vi "Move the peace.vi"(9 "Move Right":bool, 10 "Stack Array":u8[][](array[numeric]), 11 "Piece Array":u8[][](array[numeric])) -> (3 "Moved Piece Array":u8[][](array[numeric]))   [LabVIEW 2019]
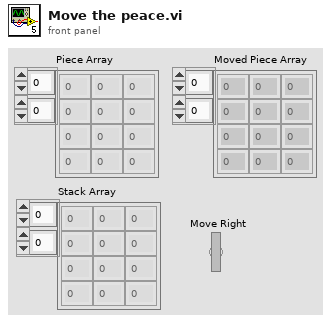
[diagram p1: front panel]
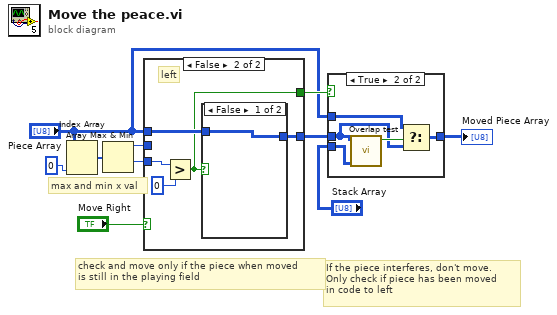
[diagram p0: block diagram]
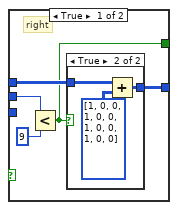
[diagram p3: hidden frame]
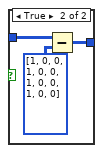
[diagram p5: hidden frame]
diagram:
  # "max and min x val"
  # "If the piece interferes, don't move.\nOnly check if piece has been moved \nin code to left"
  # "check and move only if the piece when moved\nis still in the playing field"
  n1 = Index Array(array="Piece Array", index (col)=0) -> (element=w10:u8[])  [unwired: 1 in]
  n2 = Array Max & Min(array=w10) -> (max value=w8:u8, min value=w1:u8)  [unwired: 2 out]
  n3 = case shown="False" "Move Right" {
    tunnel: w8 -> [w15 _]
    tunnel: "Piece Array" -> [w13 w23]
    tunnel: [w12 w22] -> w6
    tunnel: [w11 w21] -> w5
    tunnel: w1 -> [_ w20]
    frame True {
      # "right"
      n4 = Less?(x=w15, y=9) -> (x < y?=w12:bool)
      n5 = case shown="True" w12 {
        tunnel: w13 -> [w16 w18]
        tunnel: [w16 w17] -> w11
        frame False {
        }
        frame True {
          n6 = Add(x=w18, y=i32[][] [[1, 0, 0], [1, 0, 0], [1, 0, 0], [1, 0, 0]]) -> (x+y=w17:i32[][])
        }
      }
    }
    frame False {
      # "left"
      n7 = Greater?(x=w20, y=0) -> (0:w22:bool)
      n8 = case shown="False" w22 {
        tunnel: w23 -> [w25 w27]
        tunnel: [w25 w26] -> w21
        frame False {
        }
        frame True {
          n9 = Subtract(x=w27, y=i32[][] [[1, 0, 0], [1, 0, 0], [1, 0, 0], [1, 0, 0]]) -> (x-y=w26:i32[][])
        }
      }
    }
  }
  n10 = case shown="True" w6 {
    tunnel: w5 -> [w29 w30]
    tunnel: "Stack Array" -> [_ w31]
    tunnel: "Piece Array" -> [_ w34]
    tunnel: [w29 w33] -> w2
    frame False {
    }
    frame True {
      n11 = call "Overlap test.vi"("Stack Array"=w31, "Piece Array"=w30) -> ("Interference"=w32:bool)  [unwired: 9 in]
      n12 = Select(t=w34, s=w32, f=w30) -> (s? t:f=w33:i32[][])
    }
  }
  "Moved Piece Array" <- w2
